vi "lua_pcallk.vi"(4 "k":u64, 6 "ctx":u64, 7 "msgh":i32, 8 "error in (no error)":errorcluster, 9 "nresults":i32, 10 "nargs":i32, 11 "lua_state_p":u64) -> (0 "error out":errorcluster, 3 "lua_state_p out":u64)   [LabVIEW 2020, in "lua.dll.lvlib"]
uses:
  lua.dll.lvlib
  lua_thread_status.ctl
  lua_settop.vi
  lua54.dll
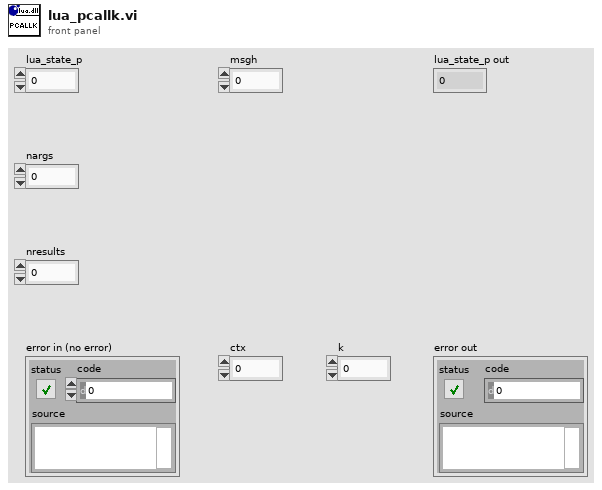
[diagram p1: front panel]
types:
  T1 = typedef "lua.dll.lvlib/lua_thread_status.ctl" = enum8{"LUA_OK", "LUA_YIELD", "LUA_ERRRUN", "LUA_ERRSYNTAX", "LUA_ERRMEM", "LUA_ERRERR"}
  T2 = typedef "lua.dll.lvlib/lua_types.ctl" = i32
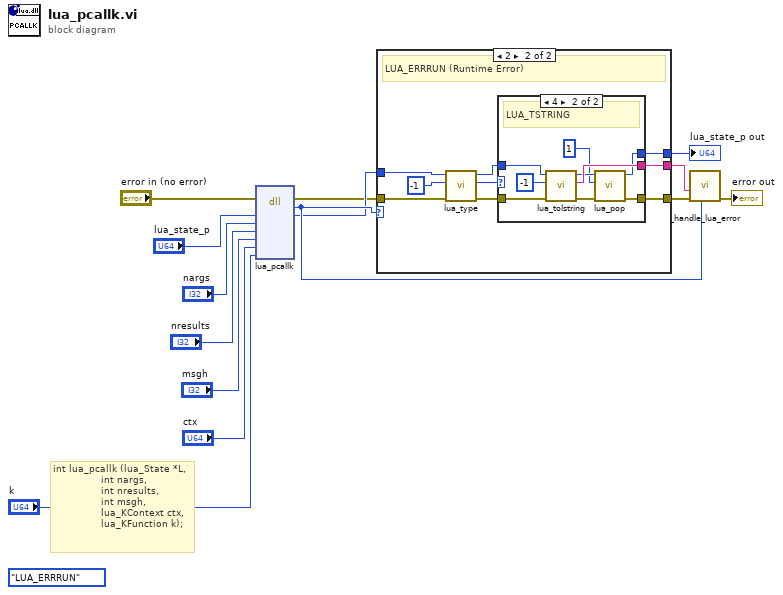
[diagram p0: block diagram]
diagram:
  (unwired) lua_thread_status."LUA_ERRRUN" ("lua status")
  # "int lua_pcallk (lua_State *L,\n                int nargs,\n                int nresults,\n                int msgh,\n                lua_KContext ctx,\n                lua_KFunction k);"
  n1 = dll-call lib="C:/Users/Nicholas Folse/Documents/workspace/github-tauterra.llc/Lua for LabVIEW/lib/lua.dll/lua54.dll" fn="lua_pcallk"(error in="error in (no error)", "lua_state_p"="lua_state_p", "nargs"="nargs", "nresults"="nresults", "msgh"="msgh", "ctx"="ctx", "k"="k") -> (error out=w2:errorcluster, "err_code"=w6:i32, "lua_state_p"=w5:u64)  [unwired: 7 in, 1 out]
  n2 = case shown="2" w6 {
    tunnel: w5 -> [w16 w22]
    tunnel: [w16 w24] -> w4
    tunnel: [_ w25] -> w3
    tunnel: w2 -> [w15 w21]
    tunnel: [w15 w23] -> w1
    frame Default {
    }
    frame 2 {
      # "LUA_ERRRUN (Runtime Error)"
      n3 = call "lua_type.vi"("error in (no error)"=w21, "index"=-1, "lua_state_p"=w22) -> ("error out"=w18:errorcluster, "lua type"=w17:T2, "lua_state_p out"=w19:u64)  [unwired: 6 in]
      n4 = case shown="4" w17 {
        tunnel: [_ w35] -> w25
        tunnel: [w27 w33] -> w24
        tunnel: [w26 w31] -> w23
        tunnel: w19 -> [w27 w29]
        tunnel: w18 -> [w26 w28]
        frame Default {
        }
        frame 4 {
          # "LUA_TSTRING"
          n5 = call "lua_tolstring.vi"("error in (no error)"=w28, "index"=-1, "lua_state_p"=w29) -> ("error out"=w32:errorcluster, "string"=w35:string, "lua_state_p out"=w34:u64)  [unwired: 6 in]
          n6 = call "lua_pop.vi"("error in (no error)"=w32, "n"=1, "lua_state_p"=w34) -> ("error out"=w31:errorcluster, "lua_state_p out"=w33:u64)  [unwired: 7 in]
        }
      }
    }
  }
  "lua_state_p out" <- w4
  n7 = call "_handle_lua_error.vi"("lua status"=w6, "error in (no error)"=w1, "error string"=w3) -> ("error out"=→"error out":errorcluster)  [unwired: 8 in]
